vi "cmd.vi"(7 "LabVIEW Web Service Request":refnum<class "Web Request.lvclass">) -> ()   [LabVIEW 2021]
uses:
  <vilib>/wsapi/Web Request.lvclass
  <userlib>/S2 Labs/Module Framework/Modules/Base/WS_Response_Cluster.ctl
  <userlib>/S2 Labs/Queued State Machine/QSM.lvclass/QSM.ctl
  <userlib>/S2 Labs/Queued State Machine/Callback Notifier/Callback Notifier.lvclass/Callback Notifier.ctl
  013b1974-e979-420a-b3f6-a5759e6721ea.vi
  1a02fae7-099a-4721-bc3d-52a14a045682.vi
  6cc4d948-7a68-4e18-81bf-1e43932b63fa.vi
  013b1974-e979-420a-b3f6-a5759e6721ea.vi/f5f13194-2e46-4b54-a6e5-ce8b0798dc89.vi
  013b1974-e979-420a-b3f6-a5759e6721ea.vi/a1053dea-4aac-46e9-b5c8-4b15c3505750.vi
  013b1974-e979-420a-b3f6-a5759e6721ea.vi/aaa66419-04fb-4bdf-8b0f-e8e43cd7e5de.vi
  <userlib>/S2 Labs/Queued State Machine/Enqueue Element.vi
  <userlib>/S2 Labs/Queued State Machine/Callback Notifier/Read Callback Notifier Ref.vi
  <userlib>/S2 Labs/Queued State Machine/Callback Notifier/Obtain Callback Notifier.vi
  <userlib>/S2 Labs/Queued State Machine/Callback Notifier/Release Reply Notifier.vi
  <vilib>/Utility/error.llb/Error Cluster From Error Code.vi
  <userlib>/S2 Labs/Error Reporting/ER Global.vi
  <userlib>/S2 Labs/Error Reporting/Error Reporting Class/subVIs/Report Error.vi
  <vilib>/JDP Science/JSONtext/Variant to JSON Text.vi
  <userlib>/S2 Labs/Queued State Machine/Callback Notifier/Callback Notifier.lvclass
  <vilib>/JDP Science/JSONtext/LVClass Serializer/JSONtext LVClass Serializer.lvclass
  <userlib>/S2 Labs/Module Framework/Modules/Base/Module.lvclass
  <userlib>/S2 Labs/Queued State Machine/QSM.lvclass
  <userlib>/S2 Labs/CVT Toolkit/CVT.lvclass
panel:
  # "Use the Web Service Request input terminal to call the VIs on the Web Services palette. Do not remove it from the connector pane unless you don't need access to the palette."
  # "Each additional control wired to the connector pane will be available as an input in the URL. To include an indicator in terminal-mode output (the default setting), it must also be wired to the connector pane."
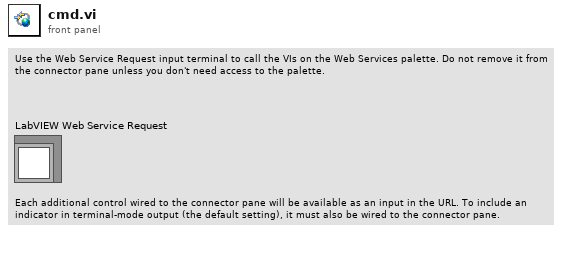
[diagram p1: front panel]
types:
  T1 = typedef "Module.lvclass/WS_Response_Cluster.ctl" = cluster{"WS Response":string, "Module Callback Response":string, "error":errorcluster}
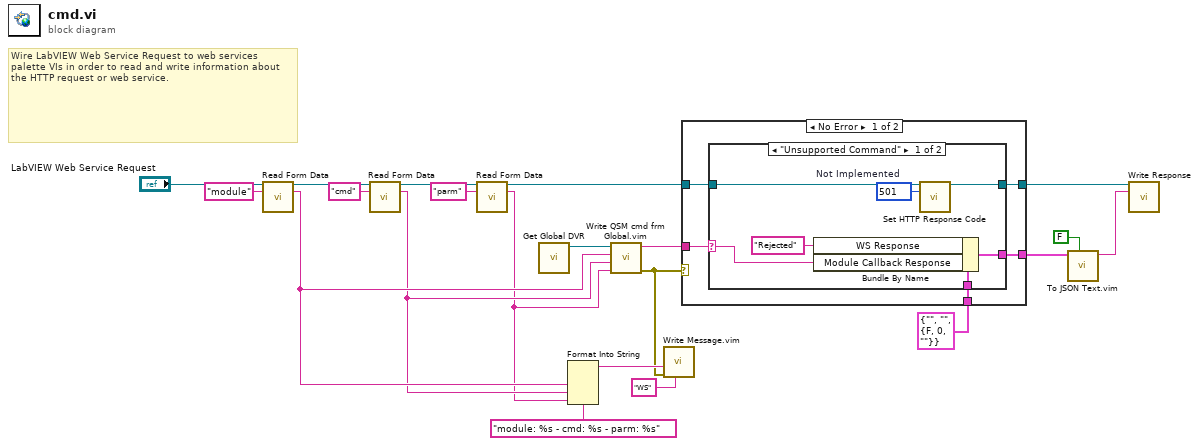
[diagram p0: block diagram]
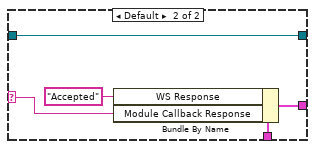
[diagram p2: hidden frame]
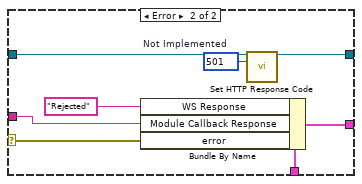
[diagram p3: hidden frame]
diagram:
  # "Wire LabVIEW Web Service Request to web services palette VIs in order to read and write information about the HTTP request or web service."
  n1 = call <vilib>:"Read Form Data.vi"("LabVIEW Web Service Request"="LabVIEW Web Service Request", "key"="module") -> ("LabVIEW Web Service Request out"=w16:refnum<class "Web Request.lvclass">, "value"=w3:string)  [unwired: 10 in, 2 out]
  n2 = call <vilib>:"Read Form Data.vi"("LabVIEW Web Service Request"=w16, "key"="cmd") -> ("LabVIEW Web Service Request out"=w15:refnum<class "Web Request.lvclass">, "value"=w2:string)  [unwired: 10 in, 2 out]
  n3 = call <vilib>:"Read Form Data.vi"("LabVIEW Web Service Request"=w15, "key"="parm") -> ("LabVIEW Web Service Request out"=w10:refnum<class "Web Request.lvclass">, "value"=w1:string)  [unwired: 10 in, 2 out]
  n4 = call <userlib>:"Get Global DVR.vi"() -> ("Global DVR"=w21:refnum<data-value>)  [unwired: 11 in]
  n5 = Format Into String(format string="module: %s - cmd: %s - parm: %s", w3, w2, w1) -> (resulting string=w14:string)  [unwired: 2 in, 1 out]
  n6 = call "Write QSM cmd frm Global.vim"("Parameter (string)"=w1, "Command"=w2, "Module"=w3, "Data Value Reference in"=w21) -> ("error out"=w11:errorcluster, "Callback Response"=w8:string)  [unwired: 6 in]
  n7 = call "Write Message.vim"("Message Tag"="WS", "error in (no error)"=w11, "Message (string)"=w14) -> ()  [unwired: 8 in, 1 out]
  n8 = case shown="No Error" w11 {
    selector: w11 -> [_ w40]
    tunnel: w10 -> [w22 w45]
    tunnel: [w23 w44] -> w9
    tunnel: w8 -> [w24 w41]
    tunnel: T1 {"WS Response"="", "Module Callback Response"="", "error"={"status"=FALSE, "code"=0, "source"=""}} -> [w26 w43]
    tunnel: [w25 w39] -> w6
    frame No Error {
      n9 = case shown="\"Unsupported Command\"" w24 {
        selector: w24 -> [w31 w35]
        tunnel: w26 -> [w33 w38]
        tunnel: [w32 w37] -> w25
        tunnel: [w28 w34] -> w23
        tunnel: w22 -> [w27 w34]
        frame "Unsupported Command" {
          w29 = 501 items=["100"=100, "101"=101, "200"=200, "201"=201, "202"=202, "203"=203, "204"=204, "205"=205, "206"=206, "300"=300, "301"=301, "302"=302, "303"=303, "304"=304, "305"=305, "306"=306, "307"=307, "400"=400, "401"=401, "402"=402, "403"=403, "404"=404, "405"=405, "406"=406, "407"=407, "408"=408, "409"=409, "410"=410, "411"=411, "412"=412, "413"=413, "414"=414, "415"=415, "416"=416, "417"=417, "500"=500, "501"=501, "502"=502, "503"=503, "504"=504, "505"=505]  # Not Implemented
          n10 = Bundle By Name(cluster=w33, "WS Response"="Rejected", "Module Callback Response"=w31) -> (w32:T1)
          n11 = call <vilib>:"Set HTTP Response Code.vi"("LabVIEW Web Service Request"=w27, "response code (200)"=w29) -> ("LabVIEW Web Service Request out"=w28:refnum<class "Web Request.lvclass">)  [unwired: 12 in, 1 out]
        }
        frame Default {
          n12 = Bundle By Name(cluster=w38, "WS Response"="Accepted", "Module Callback Response"=w35) -> (w37:T1)
        }
      }
    }
    frame Error {
      w46 = 501 items=["100"=100, "101"=101, "200"=200, "201"=201, "202"=202, "203"=203, "204"=204, "205"=205, "206"=206, "300"=300, "301"=301, "302"=302, "303"=303, "304"=304, "305"=305, "306"=306, "307"=307, "400"=400, "401"=401, "402"=402, "403"=403, "404"=404, "405"=405, "406"=406, "407"=407, "408"=408, "409"=409, "410"=410, "411"=411, "412"=412, "413"=413, "414"=414, "415"=415, "416"=416, "417"=417, "500"=500, "501"=501, "502"=502, "503"=503, "504"=504, "505"=505]  # Not Implemented
      n13 = Bundle By Name(cluster=w43, "WS Response"="Rejected", "Module Callback Response"=w41, "error"=w40) -> (w39:T1)
      n14 = call <vilib>:"Set HTTP Response Code.vi"("LabVIEW Web Service Request"=w45, "response code (200)"=w46) -> ("LabVIEW Web Service Request out"=w44:refnum<class "Web Request.lvclass">)  [unwired: 12 in, 1 out]
    }
  }
  n15 = call "To JSON Text.vim"("enable LabVIEW extensions? (T)"=FALSE, "Anything"=w6) -> ("<JSON>"=w4:string)  [unwired: 8 in, 1 out]
  n16 = call <vilib>:"Write Response.vi"("LabVIEW Web Service Request"=w9, "response string"=w4) -> ()  [unwired: 12 in, 2 out]
